vi "Update Motor Angle Setpoint.vi"(8 "error in (no error)":errorcluster, 10 "angle":dbl, 11 "motor communication in":refnum<class "NI_Robotics_Motor Communication.lvclass">) -> (0 "error out":errorcluster, 1 "failed?":bool, 3 "motor communication out":refnum<class "NI_Robotics_Motor Communication.lvclass">)   [LabVIEW 2017, in "NI_Robotics_Motor Communication.lvclass"]
uses:
  <vilib>/robotics/Actuation/Motor Communication/NI_Robotics_Motor Communication.lvclass
  <vilib>/robotics/Actuation/Motor Communication/Motor State Mode.ctl
  <vilib>/robotics/Utilities/Generate Error.vi
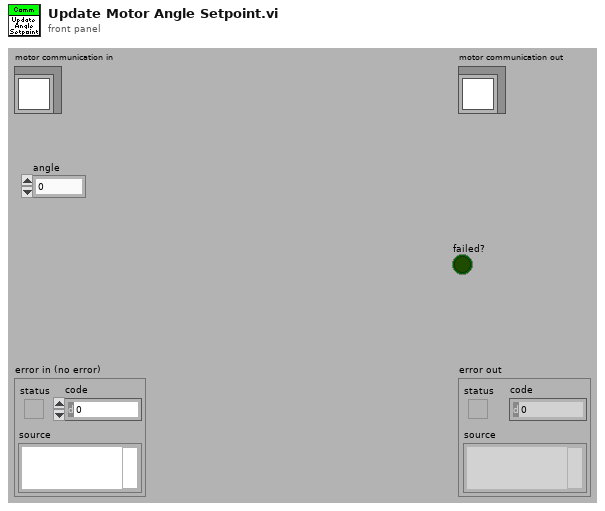
[diagram p1: front panel]
types:
  T1 = typedef "NI_Robotics_Motor Communication.lvclass/Motor State Mode.ctl" = u16
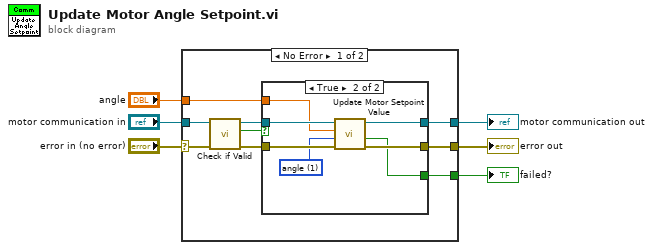
[diagram p0: block diagram]
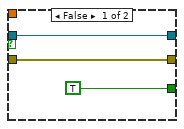
[diagram p2: hidden frame]
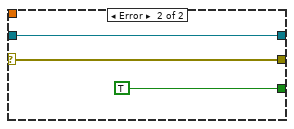
[diagram p3: hidden frame]
diagram:
  n1 = case shown="No Error" "error in (no error)" {
    selector: "error in (no error)" -> [w9 w28]
    tunnel: [w13 w28] -> w5
    tunnel: [w15 w27] -> w3
    tunnel: "motor communication in" -> [w11 w27]
    tunnel: "angle" -> [w14 _]
    tunnel: [w12 TRUE ("failed")] -> w1
    frame No Error {
      n2 = call <vilib>:"Check if Valid.vi"("error in (no error)"=w9, "motor communication in"=w11) -> ("error out"=w8:errorcluster, "valid?"=w7:bool, "motor communication out"=w10:refnum<class "NI_Robotics_Motor Communication.lvclass">)  [unwired: 7 in]
      n3 = case shown="True" w7 {
        tunnel: [w18 w25] -> w15
        tunnel: w14 -> [_ w20]
        tunnel: [w17 w24] -> w13
        tunnel: [TRUE ("failed") w23] -> w12
        tunnel: w10 -> [w18 w22]
        tunnel: w8 -> [w17 w21]
        frame False {
        }
        frame True {
          w19 = T1 1 items=["undefined", "angle", "velocity"] ("state mode")
          n4 = call-dynamic "Update Motor Setpoint Value.vi"("error in (no error)"=w21, "state mode"=w19, "value"=w20, "motor communication in"=w22) -> ("error out"=w24:errorcluster, "failed?"=w23:bool, "motor communication out"=w25:refnum<class "NI_Robotics_Motor Communication.lvclass">)  [unwired: 5 in]
        }
      }
    }
    frame Error {
    }
  }
  "error out" <- w5
  "motor communication out" <- w3
  "failed?" <- w1
